vi "FPGA_Lock-In_PID (1).vi"() -> ()   [LabVIEW 2012]
uses:
  <vilib>/FPGAPlugInAG/PCI-7831R/niLvFpga_Open_PCI-7831R.vi
  <vilib>/Utility/error.llb/Error Cluster From Error Code.vi
  <vilib>/rvi/errors/niLvFpgaAdjustHostInterfaceError.vi
  <vilib>/FPGAPlugInAG/PCI-7831R/niLvFpga_Abort_PCI-7831R.vi
  <vilib>/FPGAPlugInAG/PCI-7831R/niLvFpga_Close_PCI-7831R.vi
  <vilib>/rvi/interface/nirviOpenFPGA/nirviOpenFPGA.xnode
  SB130-XPS/Documents/FPGA-project-apporach-retraction/FPGA Bitfiles/Apporach-Retract_FPGATarget_LIAFPGA3a-PDTest_L-X5ia9B-g4.lvbitx
  Documents/FPGA PLL/LIA_FPGA3a-PD Test.vi
  <vilib>/rvi/interface/nirviReadWriteControl/nirviReadWriteControl.xnode
  <vilib>/rvi/interface/nirviMethod/nirviMethod.xnode
  <vilib>/rvi/interface/nirviCloseFPGA/nirviCloseFPGA.xnode
  NiFpgaLv.dll
panel:
  out "Ref":i32
  out "Sig":i32
  out "Reference Output":dbl
  out "P+I Error":dbl
  in  "Integral Gain":dbl
  in  "Proportional Gain":ext
  out "PID Input Error":dbl
  in  "PID Stop":bool
  out "Phase (Rad) Shift Difference":dbl
  out "Partial Phase":dbl
  out "Phase (Degree) Shift Difference":dbl
  out "P1":dbl
  out "P2":dbl
  out "Signal Output":dbl
  out "Filtered Signal":dynamicdata(graph)
  out "Multiplication of Signals":dynamicdata(graph)
  in  "Lock-In Stop":bool
  out "Freq":dbl
  out "Amp_Signal":dbl
  out "Freq":dbl
  out "Amp_Ref":dbl
  # "Reference Signal"
  # "Input Signal"
  # "PID Microcontroller"
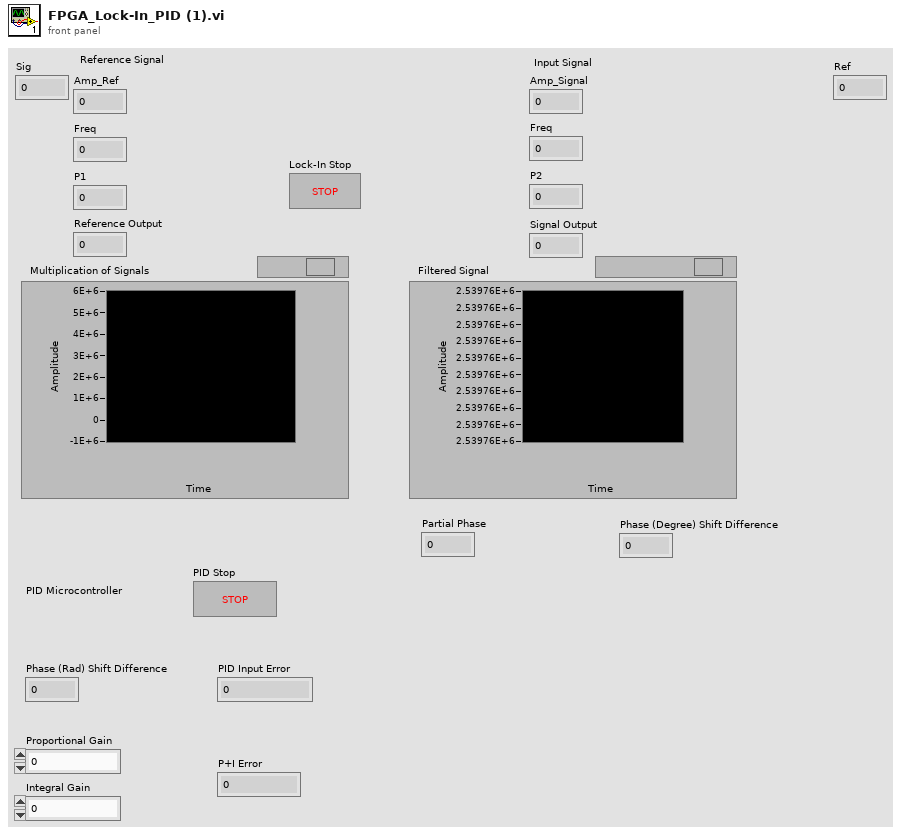
[diagram p1: front panel]
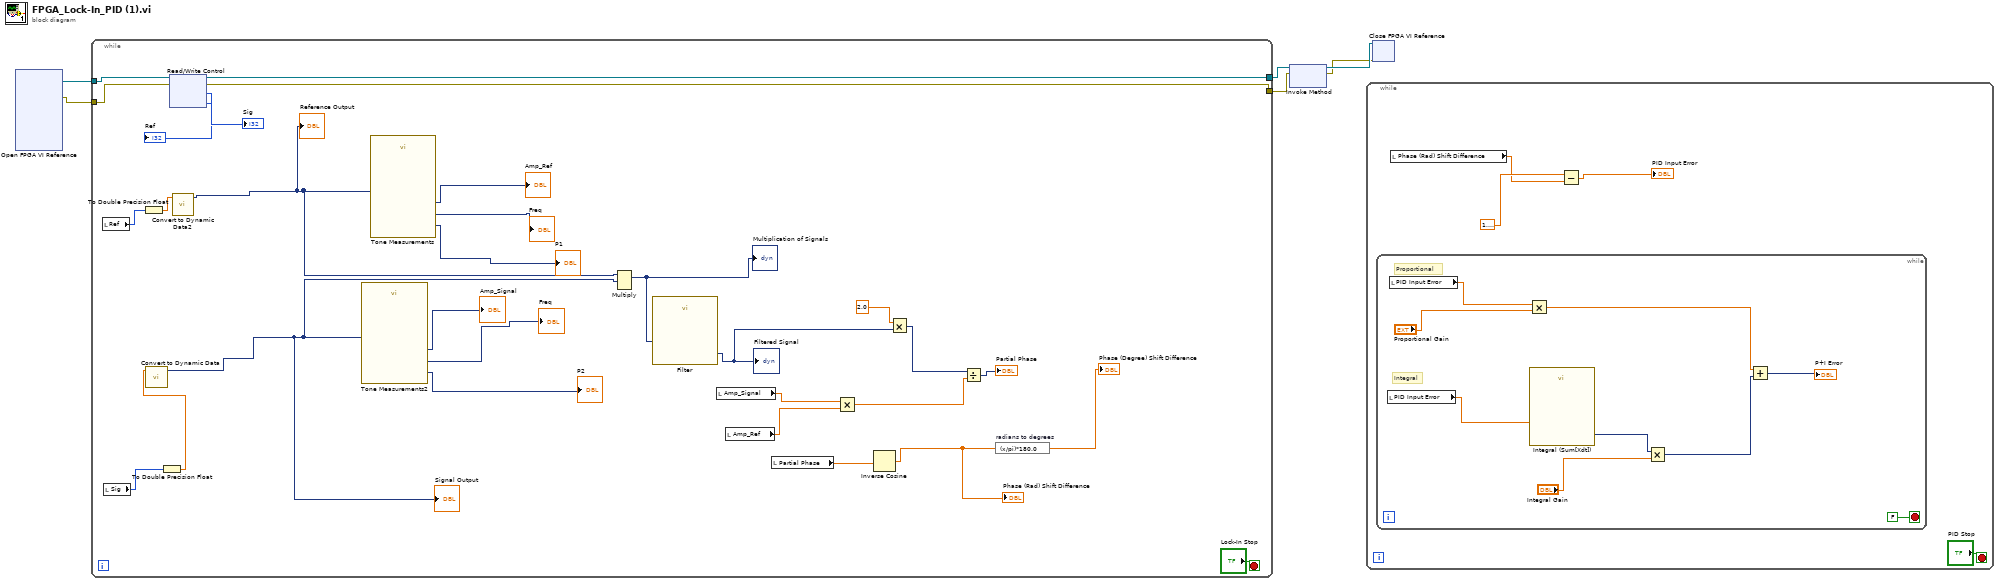
[diagram p0: block diagram]
diagram:
  n1 = xnode "Open FPGA VI Reference"() -> ("FPGA VI Reference Out"=w6:refnum<k20>, "error out"=w5:errorcluster)  [unwired: 2 in]
  n2 = while {
    tunnel: w6 -> [w16]
    tunnel: w5 -> [w15]
    tunnel: [w8] -> w4
    tunnel: [w7] -> w3
    stop <- "Lock-In Stop" stop-if-true
    n3 = local read "Ref"() -> (w11:i32)
    n4 = local read "Sig"() -> (w12:i32)
    n5 = To Double Precision Float(number=w11) -> (double precision float=w10:dbl)
    n6 = To Double Precision Float(number=w12) -> (double precision float=w9:dbl)
    n7 = call "Convert to Dynamic Data"("Double"=w9) -> ("Dynamic Data Type"=w17:dynamicdata)  [unwired: 3 in]
    "Signal Output" <- w17
    n8 = xnode "Read/Write Control"("FPGA VI Reference In"=w16, "error in"=w15) -> ("FPGA VI Reference Out"=w8:refnum<k20>, "error out"=w7:errorcluster, "sig"=→"Sig":i16, "ref"=→"Ref":i16)
    n9 = call "Convert to Dynamic Data2"("Double"=w10) -> ("Dynamic Data Type"=w18:dynamicdata)  [unwired: 3 in]
    "Reference Output" <- w18
    n10 = call "Tone Measurements2"("Signals"=w17) -> ("Phase"=→"P2":dynamicdata, "Frequency"=→"Freq":dynamicdata, "Amplitude"=→"Amp_Signal":dynamicdata)  [unwired: 7 in, 1 out]
    n11 = call "Tone Measurements"("Signals"=w18) -> ("Phase"=→"P1":dynamicdata, "Frequency"=→"Freq":dynamicdata, "Amplitude"=→"Amp_Ref":dynamicdata)  [unwired: 7 in, 1 out]
    n12 = Multiply(1:w17, 2:w18) -> (0:w31:dynamicdata)  [unwired: 1 in, 1 out]
    "Multiplication of Signals" <- w31
    n13 = call "Filter"("Signal"=w31) -> ("Filtered Signal"=w27:dynamicdata)  [unwired: 9 in, 1 out]
    "Filtered Signal" <- w27
    n14 = local read "Amp_Signal"() -> (w26:dbl)
    n15 = local read "Amp_Ref"() -> (w25:dbl)
    n16 = local read "Partial Phase"() -> (w21:dbl)
    n17 = Multiply(x=w26, y=w25) -> (x*y=w23:dbl)
    n18 = Inverse Cosine(1:w21) -> (0:w19:dbl)
    "Phase (Rad) Shift Difference" <- w19
    n19 = Multiply(x=2.0, y=w27) -> (x*y=w24:dynamicdata)
    n20 = Divide(x=w24, y=w23) -> (x/y=→"Partial Phase":dynamicdata)
    n21 = expression code="(x/pi)*180.0" "radians to degrees"(w19) -> (→"Phase (Degree) Shift Difference":dbl)
  }
  n22 = xnode "Invoke Method"("FPGA VI Reference In"=w4, "error in"=w3) -> ("FPGA VI Reference Out"=w2:refnum<k20>, "error out"=w1:errorcluster)
  n23 = while {
    stop <- "PID Stop" stop-if-true
    n24 = while {
      stop <- FALSE stop-if-true
      # "Integral"
      # "Proportional"
      n25 = local read "PID Input Error"() -> (w46:dbl)
      n26 = local read "PID Input Error"() -> (w48:dbl)
      n27 = Multiply(x=w48, y="Proportional Gain") -> (x*y=w43:ext)
      n28 = call "Integral (Sum[Xdt])"("Signals"=w46) -> ("Result"=w45:dynamicdata)  [unwired: 5 in, 1 out]
      n29 = Multiply(x=w45, y="Integral Gain") -> (x*y=w42:dynamicdata)
      n30 = Add(x=w43, y=w42) -> (x+y=→"P+I Error":dynamicdata)
    }
    n31 = local read "Phase (Rad) Shift Difference"() -> (w37:dbl)
    n32 = Subtract(x=1.5707963267948966, y=w37) -> (x-y=→"PID Input Error":dbl)
  }
  n33 = xnode "Close FPGA VI Reference"("FPGA VI Reference In"=w2, "error in"=w1) -> ()  [unwired: 1 out]
